vi "LU_20_profilometers_main__.vi"() -> ()   [LabVIEW 2015]
doc: "Профилометры ЛУ-20"
uses:
  <vilib>/NI/Modbus Library/API/Master/Modbus Master.lvclass
  <vilib>/Utility/error.llb/DialogType.ctl
panel:
  out "zLine":i32[](array[numeric])
  in  "Tab Control":enum32{"ИЗМЕРЕНИЯ", "НАСТРОЙКИ"}(tab)
  in  "Блок 2 show":bool=TRUE
  in  "Блок 1 show":bool=TRUE
  out "Изм. блок 2":dbl format="%#.2f"
  out "Изм. блок 1":dbl format="%#.2f"
  out "time":string
  out "trig led":bool
  out "Прериод, сек.":u8
  in  "Сброс":bool
  in  "Q мин. 2":dbl=-20.0 min=-200.0 max=4000.0 step=1.0
  in  "Q макс. 2":dbl=4000.0 min=0.0 max=4200.0 step=1.0
  in  "Autoscale 2":bool
  in  "IP  2":string
  in  "Порт  2":u16
  in  "ID блока 2":u8=80
  in  "Т интегрирования, мкс":u16=30 min=10 max=800 step=10
  in  "Шкала измерений":enum16{"3 пКл", "6 пКл", "12 пКл"}(ring)
  in  "stop":bool
  in  "IP":string
  in  "Порт":u16
  in  "ID блока 1":u8=80
  in  "Пароль":string
  in  "Q мин.":dbl=-100.0 min=-200.0 max=4000.0 step=1.0
  in  "Q макс.":dbl=4000.0 min=0.0 max=4200.0 step=1.0
  in  "Autoscale":bool
  in  "Уст. 0":bool
  out "empty arr":dbl[](array[numeric])
  out "Y1z":dbl[](array[numeric])
  out "X1z":dbl[](array[numeric])
  out "X2z":dbl[](array[numeric])
  out "Y2z":dbl[](array[numeric])
  out "zero lvl":dbl[](array[numeric])
  out "update graphs":bool=TRUE
  out "t2":timestamp
  in  "dev 2 upd":bool
  in  "dev 1 upd":bool
  out "Блок 2":bool
  out "X axis":i32[](array[numeric])
  out "Блок 1":bool
  out "Связь":refnum<class "Modbus Master.lvclass">
  out "X":cluster{"empty arr":dbl[], "X2":dbl[]}[](graph)=[{"empty arr"=[-10.0, -9.0, -8.0, -7.0, -6.0, -5.0, -4.0, -3.0, -2.0, -1.0, 0.0, 1.0, 2.0, 3.0, 4.0, 5.0, 6.0, 7.0, 8.0, 9.0, 10.0, 11.0, 12.0, 13.0], "X2"=[0.0, 0.0, 0.0, 0.0, 0.0, 0.0, 0.0, 0.0, 0.0, 0.0, 0.0, 0.0, 0.0, 0.0, 0.0, 0.0, 0.0, 0.0, 0.0, 0.0, 0.0, 0.0, 0.0, 0.0]}, {"empty arr"=[-10.0, -9.0, -8.0, -7.0, -6.0, -5.0, -4.0, -3.0, -2.0, -1.0, 0.0, 1.0, 2.0, 3.0, 4.0, 5.0, 6.0, 7.0, 8.0, 9.0, 10.0, 11.0, 12.0, 13.0], "X2"=[-5.0, -5.0, -2.0, -6.0, -6.0, -7.0, 5.0, -5.0, 69.0, -5.0, -6.0, -4.0, -7.0, -5.0, -5.0, -4.0, -1.0, -5.0, -1.0, -6.0, -2.0]}, {"empty arr"=[0.0, 0.0, 0.0, 0.0, 0.0, 0.0, 0.0, 0.0, 0.0, 0.0, 0.0, 0.0, 0.0, 0.0, 0.0, 0.0, 0.0, 0.0, 0.0, 0.0, 0.0, 0.0, 0.0, 0.0], "X2"=[0.0, 200.0, 400.0, 600.0, 800.0, 1000.0, 1200.0, 1400.0, 1600.0, 1800.0, 2000.0, 2200.0, 2400.0, 2600.0, 2800.0, 3000.0, 3200.0, 3400.0, 3600.0, 3800.0, 4000.0, 4200.0, 4400.0, 4600.0]}] caption="gX1"
  out "X2":dbl[](array[numeric])
  out "X1":dbl[](array[numeric])
  out "Связь 2":refnum<class "Modbus Master.lvclass">
  out "Y":cluster{"empty arr":dbl[], "Y2":dbl[]}[](graph)
  out "Y2":dbl[](array[numeric])
  out "Y1":dbl[](array[numeric])
  # "Цикл"
  # "Сумма"
  # "усл. ед."
  # "Отобразить?"
  # "усл. ед."
  # "Сумма"
  # "Отобразить?"
  # "Блок 1"
  # "Блок 2"
  # "Конфигурация изм."
  # "Шкала графика X"
  # "Шкала графика Y"
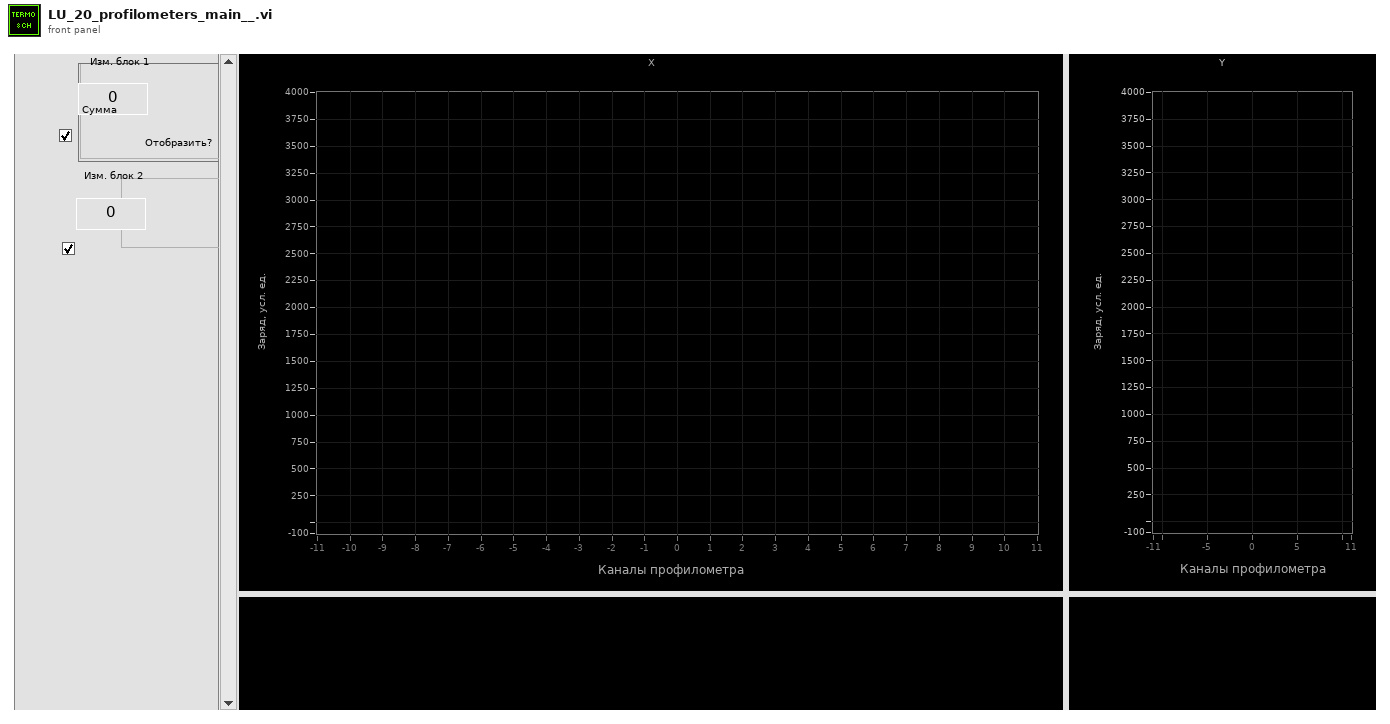
[diagram p1: front panel]
types:
  T1 = typedef "DialogType.ctl" = u16
  T2 = enum8{"Enabled", "Disabled", "Disabled and Grayed Out"}
  T3 = enum16{"open", "replace", "create", "open or create", "replace or create", "replace or create with confirmation"}
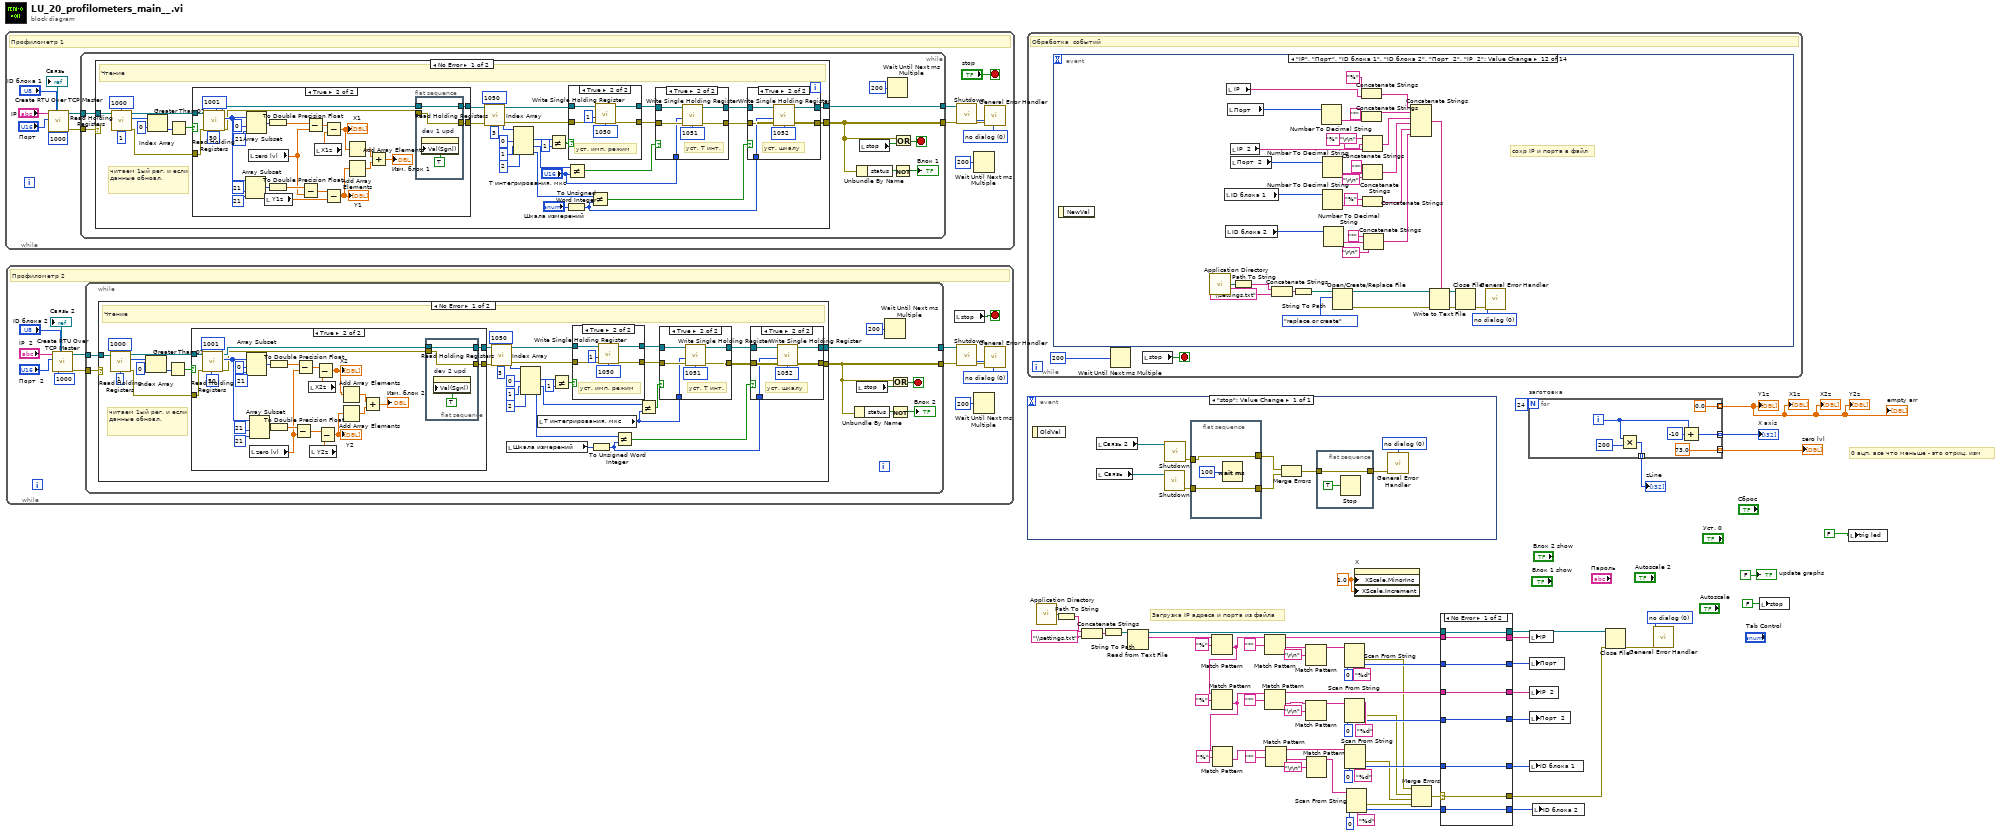
[diagram p0: block diagram]
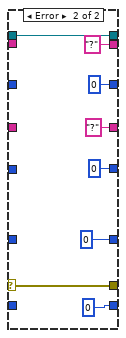
[diagram p2: hidden frame]
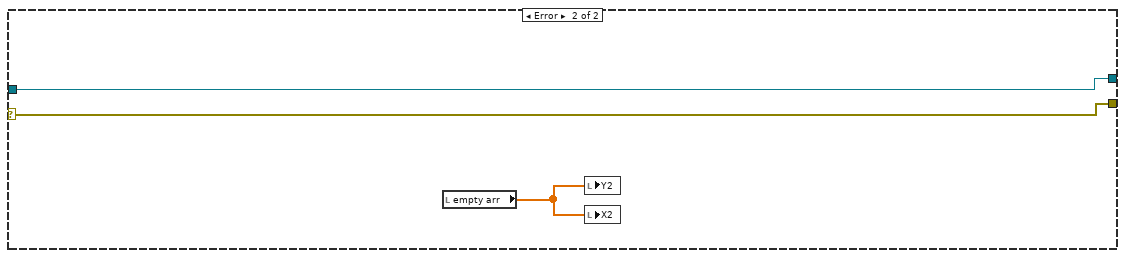
[diagram p7: hidden frame]
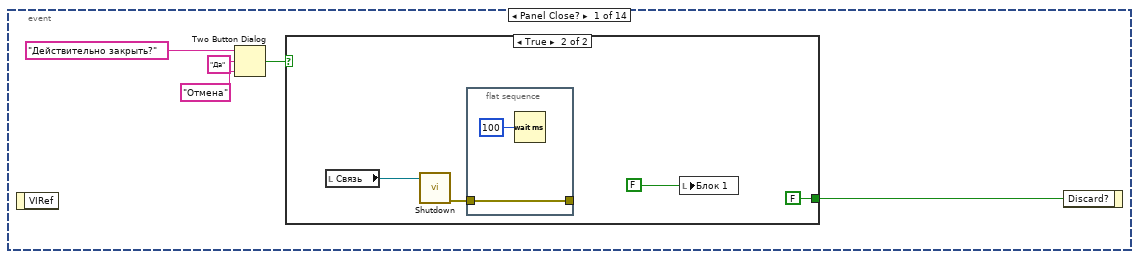
[diagram p8: hidden frame]
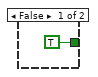
[diagram p9: hidden frame]
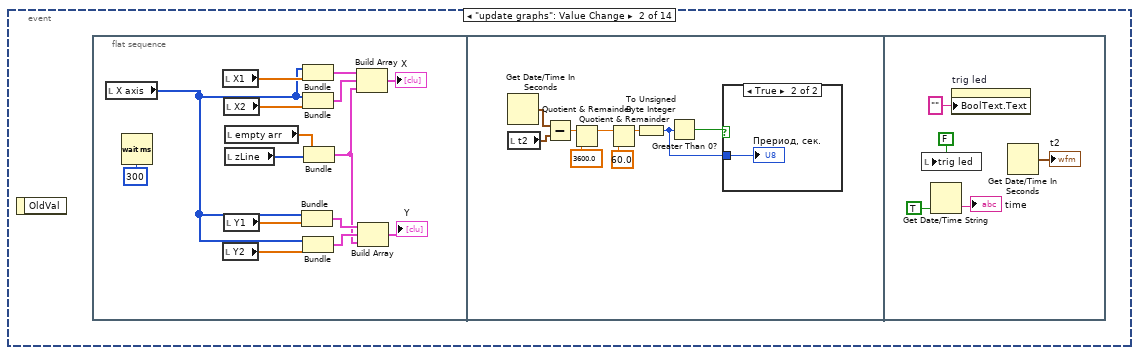
[diagram p10: hidden frame]
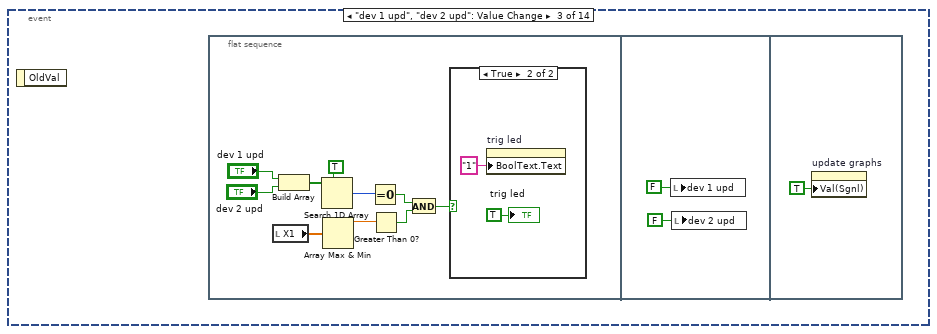
[diagram p12: hidden frame]
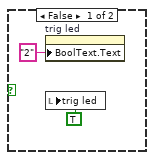
[diagram p13: hidden frame]
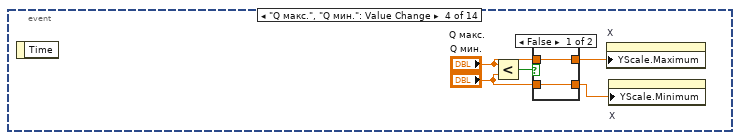
[diagram p14: hidden frame]
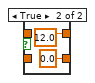
[diagram p15: hidden frame]
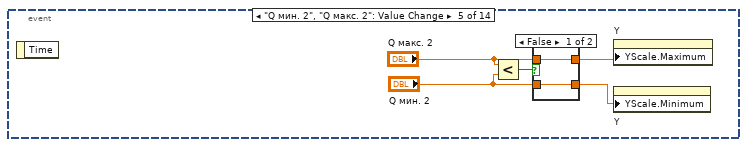
[diagram p16: hidden frame]
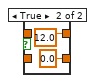
[diagram p17: hidden frame]
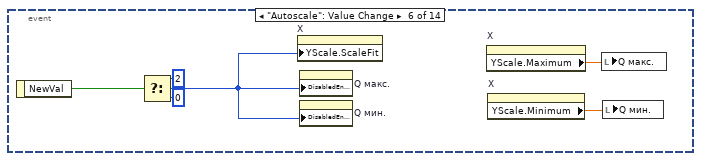
[diagram p18: hidden frame]
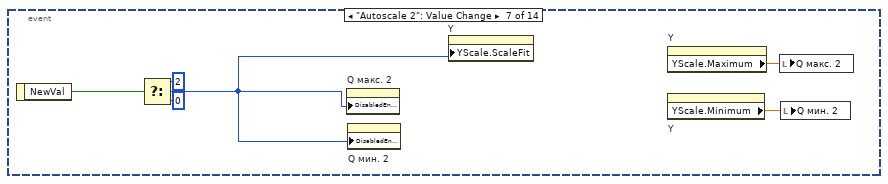
[diagram p19: hidden frame]
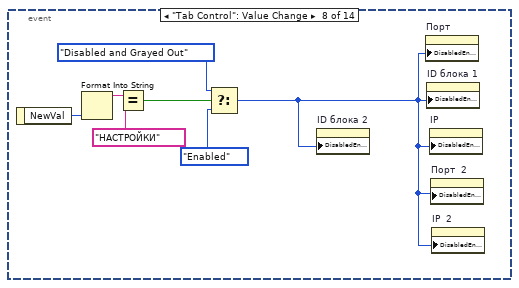
[diagram p20: hidden frame]
diagram:
  w2 = 1.0 ("X Scale.Range:Increment")
  w5 = T1 0 items=["no dialog", "OK message", "continue or stop message", "OK message + warnings", "continue/stop + warnings"] ("type of dialog (OK msg:1)")
  # "0 ацп, все что меньше - это отриц. изм"
  # "Загрузка IP адреса и порта из файла"
  n1 = while {
    stop <- "stop" stop-if-true
    w66 = T1 0 items=["no dialog", "OK message", "continue or stop message", "OK message + warnings", "continue/stop + warnings"] ("type of dialog (OK msg:1)")
    # "Профилометр 1"
    n2 = call "Create RTU Over TCP Master.vi"("unit ID"="ID блока 1", "connect timeout ms"=1000, "port (502)"="Порт", "address"="IP") -> ("error out"=w70:errorcluster, "TCP master instance"=w71:refnum<class "Modbus Master.lvclass">)  [unwired: 6 in]
    "Связь" <- w71
    n3 = while {
      tunnel: w71 -> [w85]
      tunnel: w70 -> [w84]
      tunnel: [w78] -> w69
      tunnel: [w83] -> w68
      stop <- w81 stop-if-true
      n4 = case shown="No Error" w84 {
        selector: w84 -> [_ w178]
        tunnel: w85 -> [w118 w179]
        tunnel: [w96 w178] -> w78
        tunnel: [w97 w179] -> w83
        frame No Error {
          # "читаем 1ый рег. и если данные обновл."
          # "Чтение"
          n5 = call-dynamic "Read Holding Registers.vi"("number of inputs"=u16 1, "starting address"=u16 1000, "Modbus master in"=w118) -> ("error out"=w112:errorcluster, "register values"=w117:u16[], "Modbus master out"=w113:refnum<class "Modbus Master.lvclass">)  [unwired: 6 in]
          n6 = Index Array(array=w117, index=0) -> (element=w115:u16)
          n7 = Greater Than 0?(x=w115) -> (x > 0?=w114:bool)
          n8 = case shown="True" w114 {
            tunnel: w113 -> [w146 w171]
            tunnel: w112 -> [w145 w170]
            tunnel: [w146 w158] -> w109
            tunnel: [w145 w160] -> w108
            frame False {
            }
            frame True {
              n9 = call-dynamic "Read Holding Registers.vi"("error in"=w170, "number of inputs"=u16 50, "starting address"=u16 1001, "Modbus master in"=w171) -> ("error out"=w161:errorcluster, "register values"=w164:u16[], "Modbus master out"=w159:refnum<class "Modbus Master.lvclass">)  [unwired: 5 in]
              n10 = Array Subset(array=w164, index=21, length=21) -> (w163:u16[])
              n11 = Array Subset(array=w164, index=0, length=21) -> (w167:u16[])
              n12 = local read "zero lvl"() -> (w153:dbl[])
              n13 = local read "Y1z"() -> (w162:dbl[])
              n14 = To Double Precision Float(number=w167) -> (double precision float=w157:dbl[])
              n15 = To Double Precision Float(number=w163) -> (double precision float=w154:dbl[])
              n16 = Subtract(x=w154, y=w153) -> (x-y=w155:dbl[])
              n17 = Subtract(x=w157, y=w153) -> (x-y=w156:dbl[])
              n18 = local read "X1z"() -> (w151:dbl[])
              n19 = Subtract(x=w156, y=w151) -> (x-y=w152:dbl[])
              "X1" <- w152
              n20 = Subtract(x=w155, y=w162) -> (x-y=w150:dbl[])
              "Y1" <- w150
              n21 = Add Array Elements(numeric array=w152) -> (sum=w148:dbl)
              n22 = Add Array Elements(numeric array=w150) -> (sum=w149:dbl)
              n23 = Add(x=w148, y=w149) -> (x+y=→"Изм. блок 1":dbl)
              n24 = flat-sequence {
                tunnel: w161 -> [w176]
                tunnel: [w176] -> w160
                tunnel: w159 -> [w175]
                tunnel: [w175] -> w158
                frame #0 {
                  n25 = property on="dev 1 upd" class="Bool (strict)"("Val(Sgnl)"=TRUE ("dev 1 upd")) -> ()  [unwired: 2 in, 2 out]
                }
              }
            }
          }
          n26 = call-dynamic "Read Holding Registers.vi"("error in"=w108, "number of inputs"=u16 3, "starting address"=u16 1050, "Modbus master in"=w109) -> ("error out"=w104:errorcluster, "register values"=w106:u16[], "Modbus master out"=w107:refnum<class "Modbus Master.lvclass">)  [unwired: 5 in]
          n27 = Index Array(array=w106, index #1=0 ("index"), index #2=1 ("index"), index #3=2 ("index")) -> (element #1=w110:u16, element #2=w103:u16, element #3=w94:u16)
          n28 = Not Equal?(x=w110, y=u16 1) -> (x != y?=w111:bool)
          n29 = To Unsigned Word Integer(number="Шкала измерений") -> (unsigned 16bit integer=w91:u16)
          n30 = Not Equal?(x=w103, y="Т интегрирования, мкс") -> (x != y?=w95:bool)
          n31 = case shown="True" w111 {
            tunnel: [w138 w143] -> w102
            tunnel: [w137 w142] -> w101
            tunnel: w107 -> [w138 w141]
            tunnel: w104 -> [w137 w139]
            frame False {
            }
            frame True {
              # "уст. имп. режим"
              n32 = call-dynamic "Write Single Holding Register.vi"("error in"=w139, "register to write"=u16 1, "address"=u16 1050 ("starting address"), "Modbus master in"=w141) -> ("error out"=w142:errorcluster, "Modbus master out"=w143:refnum<class "Modbus Master.lvclass">)  [unwired: 6 in]
            }
          }
          n33 = Not Equal?(x=w94, y=w91) -> (x != y?=w93:bool)
          n34 = case shown="True" w95 {
            tunnel: [w130 w135] -> w100
            tunnel: [w129 w134] -> w99
            tunnel: w102 -> [w130 w133]
            tunnel: w101 -> [w129 w132]
            tunnel: "Т интегрирования, мкс" -> [_ w131]
            frame False {
            }
            frame True {
              # "уст. Т инт."
              n35 = call-dynamic "Write Single Holding Register.vi"("error in"=w132, "register to write"=w131, "address"=u16 1051 ("starting address"), "Modbus master in"=w133) -> ("error out"=w134:errorcluster, "Modbus master out"=w135:refnum<class "Modbus Master.lvclass">)  [unwired: 6 in]
            }
          }
          n36 = case shown="True" w93 {
            tunnel: [w122 w127] -> w97
            tunnel: [w121 w126] -> w96
            tunnel: w100 -> [w122 w125]
            tunnel: w99 -> [w121 w124]
            tunnel: w91 -> [_ w123]
            frame False {
            }
            frame True {
              # "уст. шкалу"
              n37 = call-dynamic "Write Single Holding Register.vi"("error in"=w124, "register to write"=w123, "address"=u16 1052 ("starting address"), "Modbus master in"=w125) -> ("error out"=w126:errorcluster, "Modbus master out"=w127:refnum<class "Modbus Master.lvclass">)  [unwired: 6 in]
            }
          }
        }
        frame Error {
          n38 = local read "empty arr"() -> (w177:dbl[])
          n39 = local write "Y1"(w177) -> ()
          n40 = local write "X1"(w177) -> ()
        }
      }
      n41 = Unbundle By Name(w78) -> ("status"=w80:bool)
      n42 = local read "stop"() -> (w82:bool)
      n43 = Wait Until Next ms Multiple(millisecond multiple=u32 200) -> ()  [unwired: 1 out]
      n44 = Not(x=w80) -> (.not. x?=→"Блок 1":bool)
      n45 = Or(x=w78, y=w82) -> (x .or. y?=w81:bool)
    }
    n46 = call-dynamic "Shutdown.vi"("error in"=w69, "Modbus master in"=w68) -> ("error out"=w67:errorcluster)  [unwired: 9 in]
    n47 = Wait Until Next ms Multiple(millisecond multiple=u32 200) -> ()  [unwired: 1 out]
    n48 = call <vilib>:"General Error Handler.vi"("type of dialog (OK msg:1)"=w66, "error in (no error)"=w67) -> ()  [unwired: 1 in, 13 out]
  }
  n49 = while {
    stop <- w183 stop-if-true
    w184 = T1 0 items=["no dialog", "OK message", "continue or stop message", "OK message + warnings", "continue/stop + warnings"] ("type of dialog (OK msg:1)")
    # "Профилометр 2"
    n50 = call "Create RTU Over TCP Master.vi"("unit ID"="ID блока 2", "connect timeout ms"=1000, "port (502)"="Порт  2", "address"="IP  2") -> ("error out"=w188:errorcluster, "TCP master instance"=w189:refnum<class "Modbus Master.lvclass">)  [unwired: 6 in]
    "Связь 2" <- w189
    n51 = while {
      tunnel: w189 -> [w200]
      tunnel: w188 -> [w199]
      tunnel: [w194] -> w187
      tunnel: [w198] -> w186
      stop <- w197 stop-if-true
      n52 = case shown="No Error" w199 {
        selector: w199 -> [_ w293]
        tunnel: w200 -> [w233 w294]
        tunnel: [w201 w293] -> w194
        tunnel: [w202 w294] -> w198
        frame No Error {
          # "читаем 1ый рег. и если данные обновл."
          # "Чтение"
          n53 = call-dynamic "Read Holding Registers.vi"("number of inputs"=u16 1, "starting address"=u16 1000, "Modbus master in"=w233) -> ("error out"=w227:errorcluster, "register values"=w232:u16[], "Modbus master out"=w228:refnum<class "Modbus Master.lvclass">)  [unwired: 6 in]
          n54 = Index Array(array=w232, index=0) -> (element=w230:u16)
          n55 = Greater Than 0?(x=w230) -> (x > 0?=w229:bool)
          n56 = case shown="True" w229 {
            tunnel: w228 -> [w261 w286]
            tunnel: w227 -> [w260 w285]
            tunnel: [w261 w276] -> w206
            tunnel: [w260 w274] -> w205
            frame False {
            }
            frame True {
              n57 = call-dynamic "Read Holding Registers.vi"("error in"=w285, "number of inputs"=u16 50, "starting address"=u16 1001, "Modbus master in"=w286) -> ("error out"=w275:errorcluster, "register values"=w279:u16[], "Modbus master out"=w277:refnum<class "Modbus Master.lvclass">)  [unwired: 5 in]
              n58 = Array Subset(array=w279, index=0, length=21) -> (w282:u16[])
              n59 = Array Subset(array=w279, index=21, length=21) -> (w278:u16[])
              n60 = local read "zero lvl"() -> (w267:dbl[])
              n61 = To Double Precision Float(number=w282) -> (double precision float=w271:dbl[])
              n62 = To Double Precision Float(number=w278) -> (double precision float=w272:dbl[])
              n63 = Subtract(x=w272, y=w267) -> (x-y=w268:dbl[])
              n64 = Subtract(x=w271, y=w267) -> (x-y=w269:dbl[])
              n65 = local read "X2z"() -> (w270:dbl[])
              n66 = local read "Y2z"() -> (w273:dbl[])
              n67 = Subtract(x=w269, y=w270) -> (x-y=w264:dbl[])
              "X2" <- w264
              n68 = Subtract(x=w268, y=w273) -> (x-y=w263:dbl[])
              "Y2" <- w263
              n69 = Add Array Elements(numeric array=w264) -> (sum=w265:dbl)
              n70 = Add Array Elements(numeric array=w263) -> (sum=w266:dbl)
              n71 = Add(x=w265, y=w266) -> (x+y=→"Изм. блок 2":dbl)
              n72 = flat-sequence {
                tunnel: w277 -> [w291]
                tunnel: [w291] -> w276
                tunnel: w275 -> [w290]
                tunnel: [w290] -> w274
                frame #0 {
                  n73 = property on="dev 2 upd" class="Bool (strict)"("Val(Sgnl)"=TRUE ("dev 1 upd")) -> ()  [unwired: 2 in, 2 out]
                }
              }
            }
          }
          n74 = call-dynamic "Read Holding Registers.vi"("error in"=w205, "number of inputs"=u16 3, "starting address"=u16 1050, "Modbus master in"=w206) -> ("error out"=w221:errorcluster, "register values"=w223:u16[], "Modbus master out"=w224:refnum<class "Modbus Master.lvclass">)  [unwired: 5 in]
          n75 = local read "Шкала измерений"() -> (w203:enum16{"3 пКл", "6 пКл", "12 пКл"})
          n76 = Index Array(array=w223, index #1=0 ("index"), index #2=1 ("index"), index #3=2 ("index")) -> (element #1=w225:u16, element #2=w220:u16, element #3=w214:u16)
          n77 = local read "Т интегрирования, мкс"() -> (w204:u16)
          n78 = Not Equal?(x=w225, y=u16 1) -> (x != y?=w226:bool)
          n79 = case shown="True" w226 {
            tunnel: [w253 w258] -> w219
            tunnel: [w252 w257] -> w218
            tunnel: w224 -> [w253 w256]
            tunnel: w221 -> [w252 w254]
            frame False {
            }
            frame True {
              # "уст. имп. режим"
              n80 = call-dynamic "Write Single Holding Register.vi"("error in"=w254, "register to write"=u16 1, "address"=u16 1050 ("starting address"), "Modbus master in"=w256) -> ("error out"=w257:errorcluster, "Modbus master out"=w258:refnum<class "Modbus Master.lvclass">)  [unwired: 6 in]
            }
          }
          n81 = To Unsigned Word Integer(number=w203) -> (unsigned 16bit integer=w212:u16)
          n82 = Not Equal?(x=w214, y=w212) -> (x != y?=w213:bool)
          n83 = Not Equal?(x=w220, y=w204) -> (x != y?=w215:bool)
          n84 = case shown="True" w215 {
            tunnel: [w245 w250] -> w217
            tunnel: [w244 w249] -> w216
            tunnel: w219 -> [w245 w248]
            tunnel: w218 -> [w244 w247]
            tunnel: w204 -> [_ w246]
            frame False {
            }
            frame True {
              # "уст. Т инт."
              n85 = call-dynamic "Write Single Holding Register.vi"("error in"=w247, "register to write"=w246, "address"=u16 1051 ("starting address"), "Modbus master in"=w248) -> ("error out"=w249:errorcluster, "Modbus master out"=w250:refnum<class "Modbus Master.lvclass">)  [unwired: 6 in]
            }
          }
          n86 = case shown="True" w213 {
            tunnel: [w237 w242] -> w202
            tunnel: [w236 w241] -> w201
            tunnel: w217 -> [w237 w240]
            tunnel: w216 -> [w236 w239]
            tunnel: w212 -> [_ w238]
            frame False {
            }
            frame True {
              # "уст. шкалу"
              n87 = call-dynamic "Write Single Holding Register.vi"("error in"=w239, "register to write"=w238, "address"=u16 1052 ("starting address"), "Modbus master in"=w240) -> ("error out"=w241:errorcluster, "Modbus master out"=w242:refnum<class "Modbus Master.lvclass">)  [unwired: 6 in]
            }
          }
        }
        frame Error {
          n88 = local read "empty arr"() -> (w292:dbl[])
          n89 = local write "Y2"(w292) -> ()
          n90 = local write "X2"(w292) -> ()
        }
      }
      n91 = Unbundle By Name(w194) -> ("status"=w196:bool)
      n92 = local read "stop"() -> (w192:bool)
      n93 = Wait Until Next ms Multiple(millisecond multiple=u32 200) -> ()  [unwired: 1 out]
      n94 = Not(x=w196) -> (.not. x?=→"Блок 2":bool)
      n95 = Or(x=w194, y=w192) -> (x .or. y?=w197:bool)
    }
    n96 = local read "stop"() -> (w183:bool)
    n97 = call-dynamic "Shutdown.vi"("error in"=w187, "Modbus master in"=w186) -> ("error out"=w185:errorcluster)  [unwired: 9 in]
    n98 = Wait Until Next ms Multiple(millisecond multiple=u32 200) -> ()  [unwired: 1 out]
    n99 = call <vilib>:"General Error Handler.vi"("type of dialog (OK msg:1)"=w184, "error in (no error)"=w185) -> ()  [unwired: 1 in, 13 out]
  }
  n100 = while {
    stop <- w295 stop-if-true
    # "Обработка  событий"
    n101 = event shown="[11] \"IP\", \"Порт\", \"ID блока 1\", \"ID блока 2\", \"Порт  2\", \"IP  2\": Value Change" {
      selector: _ -> [_ _ _ _ _ _ _ _ _ _ _ _ _ _]
      dyn-events: _ -> [_ _ _ _ _ _ _ _ _ _ _ _ _ _]
      timeout: _ -> [_ _ _ _ _ _ _ _ _ _ _ _ _ _]
      event Panel Close? {
        n102 = event-data() -> ()  [unwired: 2 out]
        n103 = Two Button Dialog(message="Действительно закрыть?", 1:"Отмена" ("T button name (\"OK\")"), 2:"Да" ("T button name (\"OK\")")) -> (T button?=w301:bool)
        n104 = case shown="True" w301 {
          tunnel: [TRUE ("Discard?") FALSE ("Discard?")] -> w297
          frame False {
          }
          frame True {
            n105 = local read "Связь"() -> (w305:refnum<class "Modbus Master.lvclass">)
            n106 = call-dynamic "Shutdown.vi"("Modbus master in"=w305) -> ("error out"=w304:errorcluster)  [unwired: 10 in]
            n107 = flat-sequence {
              tunnel: w304 -> [w307]
              tunnel: [w307] -> _
              frame #0 {
                n108 = Wait (ms)(milliseconds to wait=u32 100) -> ()  [unwired: 1 out]
              }
            }
            n109 = local write "Блок 1"(FALSE ("Связь с блоком 4")) -> ()
          }
        }
        n110 = event-data("Discard?"=w297) -> ()  [unwired: 1 in, 1 out]
      }
      event "update graphs": Value Change {
        n111 = event-data() -> ()  [unwired: 2 out]
        n112 = flat-sequence {
          frame #0 {
            n113 = local read "X axis"() -> (w313:i32[])
            n114 = Wait (ms)(milliseconds to wait=u32 300) -> ()  [unwired: 1 out]
            n115 = local read "X1"() -> (w316:dbl[])
            n116 = local read "Y2"() -> (w320:dbl[])
            n117 = local read "X2"() -> (w312:dbl[])
            n118 = local read "Y1"() -> (w323:dbl[])
            n119 = local read "empty arr"() -> (w311:dbl[])
            n120 = local read "zLine"() -> (w310:i32[])
            n121 = Bundle("X axis"=w313, "Y1"=w323) -> (w319:cluster{"X axis":i32[], "Y1":dbl[]})  [unwired: 1 in]
            n122 = Bundle("X axis"=w313, "X1"=w316) -> (w322:cluster{"X axis":i32[], "X1":dbl[]})  [unwired: 1 in]
            n123 = Bundle("X axis"=w313, "X2"=w312) -> (w321:cluster{"X axis":i32[], "X2":dbl[]})  [unwired: 1 in]
            n124 = Bundle("X axis"=w313, "Y2"=w320) -> (w318:cluster{"X axis":i32[], "Y2":dbl[]})  [unwired: 1 in]
            n125 = Bundle("empty arr"=w311, "zLine"=w310) -> (w309:cluster{"empty arr":dbl[], "zLine":i32[]})  [unwired: 1 in]
            n126 = Build Array(w322, w321, w309) -> (→"X":cluster{"empty arr":dbl[], "X2":dbl[]}[])
            n127 = Build Array(w319, w318, w309) -> (→"Y":cluster{"empty arr":dbl[], "Y2":dbl[]}[])
          }
          frame #1 {
            n128 = Get Date/Time In Seconds() -> (seconds since 1Jan1904=w332:timestamp)
            n129 = local read "t2"() -> (w331:timestamp)
            n130 = Subtract(x=w332, y=w331) -> (x-y=w327:dbl)
            n131 = Quotient & Remainder(x=w327, y=3600.0 ("# sec/hour")) -> (x-y*floor(x/y)=w330:dbl)  [unwired: 1 out]
            n132 = Quotient & Remainder(x=w330, y=60.0 ("# sec/min")) -> (x-y*floor(x/y)=w326:dbl)  [unwired: 1 out]
            n133 = To Unsigned Byte Integer(number=w326) -> (unsigned 8bit integer=w324:u8)
            n134 = Greater Than 0?(x=w324) -> (x > 0?=w325:bool)
            n135 = case shown="True" w325 {
              tunnel: w324 -> [_ w333]
              frame False {
              }
              frame True {
                "Прериод, сек." <- w333
              }
            }
          }
          frame #2 {
            n136 = local write "trig led"(FALSE ("обновл")) -> ()
            n137 = Get Date/Time String(want seconds? (F)=TRUE) -> (time string=→"time":string)  [unwired: 2 in, 1 out]
            n138 = property on="trig led" class="Bool (strict)"("BoolText.Text"="" ("Boolean Text.Text")) -> ()  [unwired: 2 in, 2 out]
            n139 = Get Date/Time In Seconds() -> (seconds since 1Jan1904=→"t2":timestamp)
          }
        }
      }
      event "dev 1 upd", "dev 2 upd": Value Change {
        n140 = event-data() -> ()  [unwired: 2 out]
        n141 = flat-sequence {
          frame #0 {
            n142 = local read "X1"() -> (w341:dbl[])
            n143 = Build Array("dev 1 upd", "dev 2 upd") -> (w345:bool[])
            n144 = Search 1D Array(1D array=w345, element=TRUE) -> (index of element=w343:i32)  [unwired: 1 in]
            n145 = Array Max & Min(array=w341) -> (max value=w340:dbl)  [unwired: 3 out]
            n146 = Equal To 0?(x=w343) -> (x = 0?=w342:bool)
            n147 = Greater Than 0?(x=w340) -> (x > 0?=w339:bool)
            n148 = And(x=w342, y=w339) -> (x .and. y?=w348:bool)
            n149 = case shown="True" w348 {
              frame False {
                n150 = property on="trig led" class="Bool (strict)"("BoolText.Text"="2" ("Boolean Text.Text")) -> ()  [unwired: 2 in, 2 out]
                n151 = local write "trig led"(TRUE ("обновл")) -> ()
              }
              frame True {
                n152 = property on="trig led" class="Bool (strict)"("BoolText.Text"="1" ("Boolean Text.Text")) -> ()  [unwired: 2 in, 2 out]
                "trig led" <- TRUE ("обновл")
              }
            }
          }
          frame #1 {
            n153 = local write "dev 1 upd"(FALSE ("dev 1 upd")) -> ()
            n154 = local write "dev 2 upd"(FALSE ("dev 2 upd")) -> ()
          }
          frame #2 {
            n155 = property on="update graphs" class="Bool (strict)"("Val(Sgnl)"=TRUE ("update graphs")) -> ()  [unwired: 2 in, 2 out]
          }
        }
      }
      event "Q макс.", "Q мин.": Value Change {
        n156 = event-data() -> ()  [unwired: 2 out]
        n157 = Less?(x="Q макс.", y="Q мин.") -> (x < y?=w360:bool)
        n158 = case shown="False" w360 {
          tunnel: [w361 12.0 ("x+1")] -> w357
          tunnel: [w362 0.0 ("x+1")] -> w356
          tunnel: "Q макс." -> [w361 _]
          tunnel: "Q мин." -> [w362 _]
          frame False {
          }
          frame True {
          }
        }
        n159 = property on="X" class="XYGraph (strict)"("YScale.Maximum"=w357) -> ()  [unwired: 2 in, 2 out]
        n160 = property on="X" class="XYGraph (strict)"("YScale.Minimum"=w356) -> ()  [unwired: 2 in, 2 out]
      }
      event "Q мин. 2", "Q макс. 2": Value Change {
        n161 = event-data() -> ()  [unwired: 2 out]
        n162 = Less?(x="Q макс. 2", y="Q мин. 2") -> (x < y?=w369:bool)
        n163 = case shown="False" w369 {
          tunnel: [w370 12.0 ("x+1")] -> w368
          tunnel: [w371 0.0 ("x+1")] -> w367
          tunnel: "Q макс. 2" -> [w370 _]
          tunnel: "Q мин. 2" -> [w371 _]
          frame False {
          }
          frame True {
          }
        }
        n164 = property on="Y" class="XYGraph (strict)"("YScale.Maximum"=w368) -> ()  [unwired: 2 in, 2 out]
        n165 = property on="Y" class="XYGraph (strict)"("YScale.Minimum"=w367) -> ()  [unwired: 2 in, 2 out]
      }
      event "Autoscale": Value Change {
        n166 = event-data() -> ("NewVal"=w377:bool)  [unwired: 1 out]
        n167 = Select(t=u8 2 ("Y Scale.Scale Fit"), s=w377, f=u8 0 ("Y Scale.Scale Fit")) -> (s? t:f=w376:u8)
        n168 = property on="X" class="XYGraph (strict)"("YScale.ScaleFit"=w376) -> ()  [unwired: 2 in, 2 out]
        n169 = property on="Q макс." class="DigNum (strict)"("DisabledEnum"=w376) -> ()  [unwired: 2 in, 2 out]
        n170 = property on="Q мин." class="DigNum (strict)"("DisabledEnum"=w376) -> ()  [unwired: 2 in, 2 out]
        n171 = property on="X" class="XYGraph (strict)"() -> ("YScale.Maximum"=w375:dbl)  [unwired: 2 in, 2 out]
        n172 = property on="X" class="XYGraph (strict)"() -> ("YScale.Minimum"=w374:dbl)  [unwired: 2 in, 2 out]
        n173 = local write "Q макс."(w375) -> ()
        n174 = local write "Q мин."(w374) -> ()
      }
      event "Autoscale 2": Value Change {
        n175 = event-data() -> ("NewVal"=w383:bool)  [unwired: 1 out]
        n176 = Select(t=u8 2 ("Y Scale.Scale Fit"), s=w383, f=u8 0 ("Y Scale.Scale Fit")) -> (s? t:f=w380:u8)
        n177 = property on="Q макс. 2" class="DigNum (strict)"("DisabledEnum"=w380) -> ()  [unwired: 2 in, 2 out]
        n178 = property on="Q мин. 2" class="DigNum (strict)"("DisabledEnum"=w380) -> ()  [unwired: 2 in, 2 out]
        n179 = property on="Y" class="XYGraph (strict)"("YScale.ScaleFit"=w380) -> ()  [unwired: 2 in, 2 out]
        n180 = property on="Y" class="XYGraph (strict)"() -> ("YScale.Maximum"=w382:dbl)  [unwired: 2 in, 2 out]
        n181 = property on="Y" class="XYGraph (strict)"() -> ("YScale.Minimum"=w381:dbl)  [unwired: 2 in, 2 out]
        n182 = local write "Q макс. 2"(w382) -> ()
        n183 = local write "Q мин. 2"(w381) -> ()
      }
      event "Tab Control": Value Change {
        n184 = event-data() -> ("NewVal"=w392:enum32{"ИЗМЕРЕНИЯ", "НАСТРОЙКИ"})  [unwired: 1 out]
        n185 = Format Into String(w392) -> (resulting string=w391:string)  [unwired: 3 in, 1 out]
        n186 = Equal?(x=w391, y="НАСТРОЙКИ") -> (x = y?=w389:bool)
        n187 = Select(t=T2."Disabled and Grayed Out" ("Disabled"), s=w389, f=T2."Enabled" ("Disabled")) -> (s? t:f=w386:T2)
        n188 = property on="ID блока 2" class="DigNum (strict)"("DisabledEnum"=w386) -> ()  [unwired: 2 in, 2 out]
        n189 = property on="Порт" class="DigNum (strict)"("DisabledEnum"=w386) -> ()  [unwired: 2 in, 2 out]
        n190 = property on="ID блока 1" class="DigNum (strict)"("DisabledEnum"=w386) -> ()  [unwired: 2 in, 2 out]
        n191 = property on="IP" class="Str"("DisabledEnum"=w386) -> ()  [unwired: 2 in, 2 out]
        n192 = property on="Порт  2" class="DigNum (strict)"("DisabledEnum"=w386) -> ()  [unwired: 2 in, 2 out]
        n193 = property on="IP  2" class="Str"("DisabledEnum"=w386) -> ()  [unwired: 2 in, 2 out]
      }
      event "Пароль": Value Change {
        n194 = event-data() -> ("NewVal"=w394:string)  [unwired: 1 out]
        n195 = Equal?(x=w394, y="lu20") -> (x = y?=w393:bool)
        n196 = case shown="True" w393 {
          frame False {
          }
          frame True {
            w396 = T2."Enabled" ("Disabled")
            n197 = property on="ID блока 2" class="DigNum (strict)"("DisabledEnum"=w396) -> ()  [unwired: 2 in, 2 out]
            n198 = property on="Порт  2" class="DigNum (strict)"("DisabledEnum"=w396) -> ()  [unwired: 2 in, 2 out]
            n199 = property on="IP  2" class="Str"("DisabledEnum"=w396) -> ()  [unwired: 2 in, 2 out]
            n200 = property on="Порт" class="DigNum (strict)"("DisabledEnum"=w396) -> ()  [unwired: 2 in, 2 out]
            n201 = property on="ID блока 1" class="DigNum (strict)"("DisabledEnum"=w396) -> ()  [unwired: 2 in, 2 out]
            n202 = property on="IP" class="Str"("DisabledEnum"=w396) -> ()  [unwired: 2 in, 2 out]
            n203 = property on="Пароль" class="Str"("Value"="" ("Пароль")) -> ()  [unwired: 2 in, 2 out]
          }
        }
      }
      event "Уст. 0": Value Change {
        n204 = event-data() -> ()  [unwired: 2 out]
        n205 = local write "Уст. 0"(FALSE ("Уст. 0")) -> ()
        n206 = local read "X1"() -> (w401:dbl[])
        n207 = local read "X2"() -> (w398:dbl[])
        n208 = local read "Y1"() -> (w400:dbl[])
        n209 = local read "Y2"() -> (w399:dbl[])
        n210 = local write "X1z"(w401) -> ()
        n211 = local write "X2z"(w398) -> ()
        n212 = local write "Y1z"(w400) -> ()
        n213 = local write "Y2z"(w399) -> ()
      }
      event "Сброс": Value Change {
        n214 = event-data() -> ()  [unwired: 2 out]
        n215 = local write "Сброс"(FALSE ("Уст. 0")) -> ()
        n216 = local read "empty arr"() -> (w403:dbl[])
        n217 = local write "X1z"(w403) -> ()
        n218 = local write "X2z"(w403) -> ()
        n219 = local write "Y1z"(w403) -> ()
        n220 = local write "Y2z"(w403) -> ()
      }
      event "IP", "Порт", "ID блока 1", "ID блока 2", "Порт  2", "IP  2": Value Change {
        w437 = T1 0 items=["no dialog", "OK message", "continue or stop message", "OK message + warnings", "continue/stop + warnings"] ("type of dialog (OK msg:1)")
        # "сохр IP и порта в файл"
        n221 = event-data() -> ()  [unwired: 2 out]
        n222 = call <vilib>:"Application Directory.vi"() -> ("Application Directory"=w429:path)
        n223 = local read "ID блока 1"() -> (w415:u8)
        n224 = local read "ID блока 2"() -> (w410:u8)
        n225 = local read "IP"() -> (w421:string)
        n226 = local read "Порт"() -> (w420:u16)
        n227 = local read "IP  2"() -> (w419:string)
        n228 = local read "Порт  2"() -> (w418:u16)
        n229 = Path To String(path=w429) -> (string=w426:string)
        n230 = Concatenate Strings(w426, "\\settings.txt" ("prompt (Open existing file)")) -> (w428:string)
        n231 = String To Path(string=w428) -> (path=w425:path)
        n232 = Number To Decimal String(number=w420) -> (decimal integer string=w433:string)  [unwired: 1 in]
        n233 = Number To Decimal String(number=w418) -> (decimal integer string=w440:string)  [unwired: 1 in]
        n234 = Number To Decimal String(number=w415) -> (decimal integer string=w413:string)  [unwired: 1 in]
        n235 = Number To Decimal String(number=w410) -> (decimal integer string=w412:string)  [unwired: 1 in]
        n236 = Open/Create/Replace File(file path (use dialog)=w425, operation (0:open)=T3."replace or create") -> (refnum out=w423:refnum<file>, error out=w424:errorcluster)  [unwired: 2 in, 3 out]
        n237 = Concatenate Strings("%" ("string"), w421) -> (w432:string)
        n238 = Concatenate Strings("*" ("string"), w433) -> (w431:string)
        n239 = Concatenate Strings("\r\n", "%" ("string"), w419) -> (w441:string)
        n240 = Concatenate Strings("*" ("string"), w440, "\r\n") -> (w442:string)
        n241 = Concatenate Strings("%" ("string"), w413) -> (w408:string)
        n242 = Concatenate Strings("*" ("string"), w412, "\r\n") -> (w407:string)
        n243 = Concatenate Strings(w432, w431, w441, w442, w408, w407) -> (w430:string)
        n244 = Write to Text File(file (use dialog)=w423, text=w430, error in=w424) -> (refnum out=w435:refnum<file>, error out=w436:errorcluster)  [unwired: 2 out]
        n245 = Close File(refnum=w435, error in=w436) -> (error out=w438:errorcluster)  [unwired: 1 out]
        n246 = call <vilib>:"General Error Handler.vi"("type of dialog (OK msg:1)"=w437, "error in (no error)"=w438) -> ()  [unwired: 1 in, 13 out]
      }
      event "Блок 1 show": Value Change {
        n247 = event-data() -> ("NewVal"=w443:bool)  [unwired: 1 out]
        n248 = property on="X" class="XYGraph (strict)"("Active Plot"=u32 0) -> (error out=w445:errorcluster)  [unwired: 2 in, 1 out]
        n249 = property on="X" class="XYGraph (strict)"(error in=w445, "Plot.Visible?"=w443) -> (error out=w446:errorcluster)  [unwired: 1 in, 1 out]
        n250 = property on="Y" class="XYGraph (strict)"(error in=w446, "Active Plot"=u32 0) -> (error out=w448:errorcluster)  [unwired: 1 in, 1 out]
        n251 = property on="Y" class="XYGraph (strict)"(error in=w448, "Plot.Visible?"=w443) -> ()  [unwired: 1 in, 2 out]
      }
      event "Блок 2 show": Value Change {
        n252 = event-data() -> ("NewVal"=w449:bool)  [unwired: 1 out]
        n253 = property on="X" class="XYGraph (strict)"("Active Plot"=u32 1) -> (error out=w451:errorcluster)  [unwired: 2 in, 1 out]
        n254 = property on="X" class="XYGraph (strict)"(error in=w451, "Plot.Visible?"=w449) -> (error out=w452:errorcluster)  [unwired: 1 in, 1 out]
        n255 = property on="Y" class="XYGraph (strict)"(error in=w452, "Active Plot"=u32 1) -> (error out=w454:errorcluster)  [unwired: 1 in, 1 out]
        n256 = property on="Y" class="XYGraph (strict)"(error in=w454, "Plot.Visible?"=w449) -> ()  [unwired: 1 in, 2 out]
      }
    }
    n257 = Wait Until Next ms Multiple(millisecond multiple=u32 200) -> ()  [unwired: 1 out]
    n258 = local read "stop"() -> (w295:bool)
  }
  n259 = event shown="[0] \"stop\": Value Change" {
    selector: _ -> [_]
    dyn-events: _ -> [_]
    timeout: _ -> [_]
    event "stop": Value Change {
      w461 = T1 0 items=["no dialog", "OK message", "continue or stop message", "OK message + warnings", "continue/stop + warnings"] ("type of dialog (OK msg:1)")
      n260 = event-data() -> ()  [unwired: 1 in, 1 out]
      n261 = local read "Связь 2"() -> (w459:refnum<class "Modbus Master.lvclass">)
      n262 = local read "Связь"() -> (w463:refnum<class "Modbus Master.lvclass">)
      n263 = call-dynamic "Shutdown.vi"("Modbus master in"=w463) -> ("error out"=w462:errorcluster)  [unwired: 10 in]
      n264 = call-dynamic "Shutdown.vi"("Modbus master in"=w459) -> ("error out"=w455:errorcluster)  [unwired: 10 in]
      n265 = flat-sequence {
        tunnel: w462 -> [w467]
        tunnel: [w467] -> w457
        tunnel: [w466] -> w456
        tunnel: w455 -> [w466]
        frame #0 {
          n266 = Wait (ms)(milliseconds to wait=u32 100) -> ()  [unwired: 1 out]
        }
      }
      n267 = Merge Errors(w456, w457) -> (w458:errorcluster)
      n268 = flat-sequence {
        tunnel: w458 -> [w465]
        tunnel: [w465] -> w460
        frame #0 {
          n269 = Stop(stop? (T)=TRUE) -> ()
        }
      }
      n270 = call <vilib>:"General Error Handler.vi"("error in (no error)"=w460, "[exception action] (none:0)"=w461) -> ()  [unwired: 2 in, 12 out]
    }
  }
  n271 = call <vilib>:"Application Directory.vi"() -> ("Application Directory"=w45:path)
  n272 = Path To String(path=w45) -> (string=w44:string)
  n273 = Concatenate Strings(w44, "\\settings.txt" ("prompt (Open existing file)")) -> (w43:string)
  n274 = String To Path(string=w43) -> (path=w41:path)
  n275 = Read from Text File(file (use dialog)=w41) -> (refnum out=w53:refnum<file>, text=w39:string)  [unwired: 3 in, 2 out]
  n276 = Match Pattern(string=w39, regular expression="%") -> (after substring=w20:string)  [unwired: 1 in, 3 out]
  n277 = Match Pattern(string=w20, regular expression="%") -> (after substring=w6:string)  [unwired: 1 in, 3 out]
  n278 = Match Pattern(string=w6, regular expression="%") -> (after substring=w18:string)  [unwired: 1 in, 3 out]
  n279 = Match Pattern(string=w20, regular expression="*" ("string")) -> (before substring=w46:string, after substring=w21:string)  [unwired: 1 in, 2 out]
  n280 = Match Pattern(string=w6, regular expression="*" ("string")) -> (before substring=w28:string, after substring=w22:string)  [unwired: 1 in, 2 out]
  n281 = Match Pattern(string=w18, regular expression="*" ("string")) -> (before substring=w15:string, after substring=w7:string)  [unwired: 1 in, 2 out]
  n282 = Match Pattern(string=w21, regular expression="\r\n") -> (before substring=w36:string)  [unwired: 1 in, 3 out]
  n283 = Match Pattern(string=w22, regular expression="\r\n") -> (before substring=w33:string)  [unwired: 1 in, 3 out]
  n284 = Match Pattern(string=w7, regular expression="\r\n") -> (before substring=w8:string)  [unwired: 1 in, 3 out]
  n285 = Scan From String(format string="%d", input string=w36, default 1=u16 0 ("default value 1")) -> (error out=w24:errorcluster, output 1=w47:u16)  [unwired: 2 in, 2 out]
  n286 = Scan From String(format string="%d", input string=w33, default 1=u16 0 ("default value 1")) -> (error out=w23:errorcluster, output 1=w27:u16)  [unwired: 2 in, 2 out]
  n287 = Scan From String(format string="%d", input string=w15, default 1=u8 0 ("default value 1")) -> (error out=w10:errorcluster, output 1=w26:u8)  [unwired: 2 in, 2 out]
  n288 = Scan From String(format string="%d", input string=w8, default 1=u8 0 ("default value 1")) -> (error out=w9:errorcluster, output 1=w25:u8)  [unwired: 2 in, 2 out]
  n289 = property on="X" class="XYGraph (strict)"("XScale.MinorInc"=w2, "XScale.Increment"=w2) -> ()  [unwired: 2 in, 2 out]
  n290 = Merge Errors(w24, w23, w10, w9) -> (w48:errorcluster)
  n291 = case shown="No Error" w48 {
    selector: w48 -> [w472 w479]
    tunnel: w46 -> [w476 _]
    tunnel: w47 -> [w475 _]
    tunnel: w28 -> [w474 _]
    tunnel: w27 -> [w473 _]
    tunnel: [w476 "?"] -> w49
    tunnel: [w475 u16 0 ("default value 1")] -> w50
    tunnel: [w474 "?"] -> w51
    tunnel: [w473 u16 0 ("default value 1")] -> w52
    tunnel: w53 -> [w471 w480]
    tunnel: [w471 w480] -> w54
    tunnel: [w472 w479] -> w55
    tunnel: w26 -> [w470 _]
    tunnel: [w470 u8 0 ("default value 1")] -> w38
    tunnel: w25 -> [w469 _]
    tunnel: [w469 u8 0 ("default value 1")] -> w37
    frame No Error {
    }
    frame Error {
    }
  }
  n292 = for "заготовка" {
    N: 24 -> [_]
    tunnel: [w490] -> w62 mode=indexing
    tunnel: [0.0] -> w61 mode=indexing
    tunnel: [73.0] -> w4 mode=indexing
    tunnel: [w485] -> w1 mode=indexing
    i -> [w487]
    n293 = Multiply(x=w487, y=200) -> (x*y=w485:i32)
    n294 = Add(x=-10, y=w487) -> (x+y=w490:i32)
  }
  "X axis" <- w62
  "X1z" <- w61
  "Y1z" <- w61
  "X2z" <- w61
  "Y2z" <- w61
  "empty arr" <- w61
  "zero lvl" <- w4
  "zLine" <- w1
  n295 = local write "IP"(w49) -> ()
  n296 = local write "Порт"(w50) -> ()
  n297 = local write "IP  2"(w51) -> ()
  n298 = local write "Порт  2"(w52) -> ()
  n299 = local write "ID блока 1"(w38) -> ()
  n300 = local write "ID блока 2"(w37) -> ()
  n301 = Close File(refnum=w54, error in=w55) -> (error out=w56:errorcluster)  [unwired: 1 out]
  n302 = call <vilib>:"General Error Handler.vi"("type of dialog (OK msg:1)"=w5, "error in (no error)"=w56) -> ()  [unwired: 1 in, 13 out]
  n303 = local write "stop"(FALSE ("Boolean")) -> ()
  n304 = local write "trig led"(FALSE ("обновл")) -> ()
  "update graphs" <- FALSE ("обновл")
